vi "mqttCmdCreate.vi"(8 "error in (no error)":errorcluster, 10 "mqtt instance":refnum<class "mqtt.lvclass">) -> (0 "error out":errorcluster, 3 "mqttCmdDisconnect out":refnum<class "mqttCmdDisconnect.lvclass">)   [LabVIEW 2020, in "mqttCmdDisconnect.lvclass"]
uses:
  mqttCmdDisconnect.lvclass
  C:/Projects/Libraries/Gore SM 2020/mqtt-LabVIEW/src/class/mqtt/mqttCmd/mqttCmd.lvclass
  mqtt.lvclass
  mqttTypedef/mqttQOSlevel.ctl
  mqttTypedef/mqttMessageType.ctl
  mqttCmd.lvclass/mqttCmd.ctl
  Properties/Write Datagram.vi
  mqttCmd.lvclass
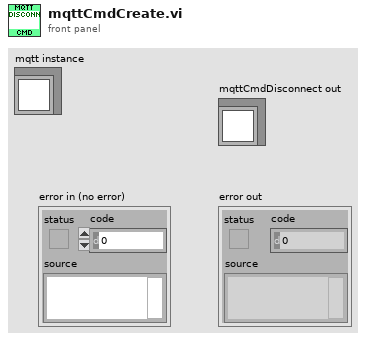
[diagram p1: front panel]
types:
  T1 = typedef "mqtt.lvclass/mqttMessageType.ctl" = enum32{"Reserved", "CONNECT", "CONNACK", "PUBLISH", "PUBACK", "PUBREC", "PUBREL", "PUBCOMP", "SUBSCRIBE", "SUBACK", "UNSUBSCRIBE", "UNSUBACK", "PINGREQ", "PINGRESP", "DISCONNECT", "Reserved2"}
  T2 = typedef "mqtt.lvclass/mqttQOSlevel.ctl" = enum8{"At most once", "At least once", "Exactly once", "Reserved"}
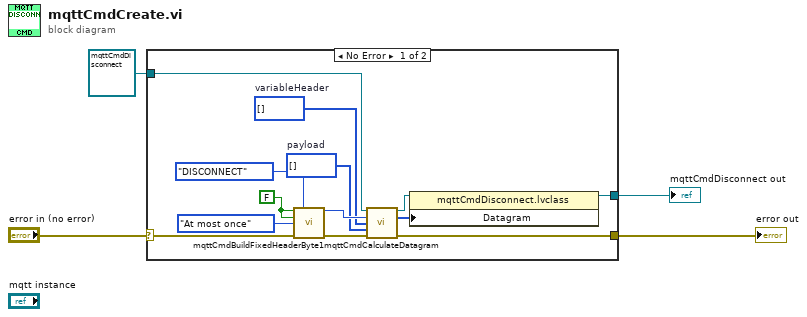
[diagram p0: block diagram]
diagram:
  n1 = case shown="No Error" "error in (no error)" {
    selector: "error in (no error)" -> [w13 w19]
    tunnel: [w5 w19] -> w3
    tunnel: [w14 w18] -> w2
    tunnel: refnum<class "mqttCmdDisconnect.lvclass"> refnum ("mqttCmdDisconnect out") -> [w12 w18]
    frame No Error {
      w8 = u8[] []  # payload
      w9 = u8[] []  # variableHeader
      w16 = FALSE
      n2 = call "mqttCmdBuildFixedHeaderByte1.vi"("retain(F)"=w16, "MessageType"=mqttMessageType."DISCONNECT", "duplicate(F)"=w16, "QoS (At most once)"=mqttQOSlevel."At most once", "error in (no error)"=w13) -> ("byte1"=w10:u8, "error out"=w7:errorcluster)  [unwired: 9 in]
      n3 = call-dynamic "mqttCmdCalculateDatagram.vi"("mqttCmd in"=w12, "FixedHeaderByte1"=w10, "variableHeader"=w9, "payload"=w8, "error in (no error)"=w7) -> ("mqttCmd out"=w11:refnum<class "mqttCmdDisconnect.lvclass">, "Datagram"=w6:u8[], "error out"=w5:errorcluster)  [unwired: 8 in]
      n4 = property class="mqttCmdDisconnect.lvclass"(reference=w11, "Datagram"=w6) -> (reference out=w14:refnum<class "mqttCmdDisconnect.lvclass">)  [unwired: 1 in, 1 out]
    }
    frame Error {
    }
  }
  "error out" <- w3
  "mqttCmdDisconnect out" <- w2
